vi "dialog_box for calibration.vi"(8 "error in (no error)":errorcluster caption="错误输入（无错误）") -> (0 "error out":errorcluster caption="错误输出", 2 "parameter for calibration out":T1, 3 "Cancelled?":bool caption="取消？")   [LabVIEW 2017]
doc: "该模板用于创建能够进行事件处理的对话框。"
uses:
  parameter set for calibration.ctl
panel:
  in  "磁铁位置":dbl=3.5
  in  "磁球大小（直径）":dbl=1.0
  in  "parameter for calibration":T1
  in  "校准步数":i32=20
  in  "首尾等待时间(s)":u32=1 caption="首尾I{卂时间(s)"
  in  "每步采样（frame）":u32=200
  in  "校准步长":dbl=0.1
  in  "分子长度（um）":dbl=1.0
  in  "Cancel":bool caption="取消"
  in  "OK":bool caption="确定"
  # "校准参数设置"
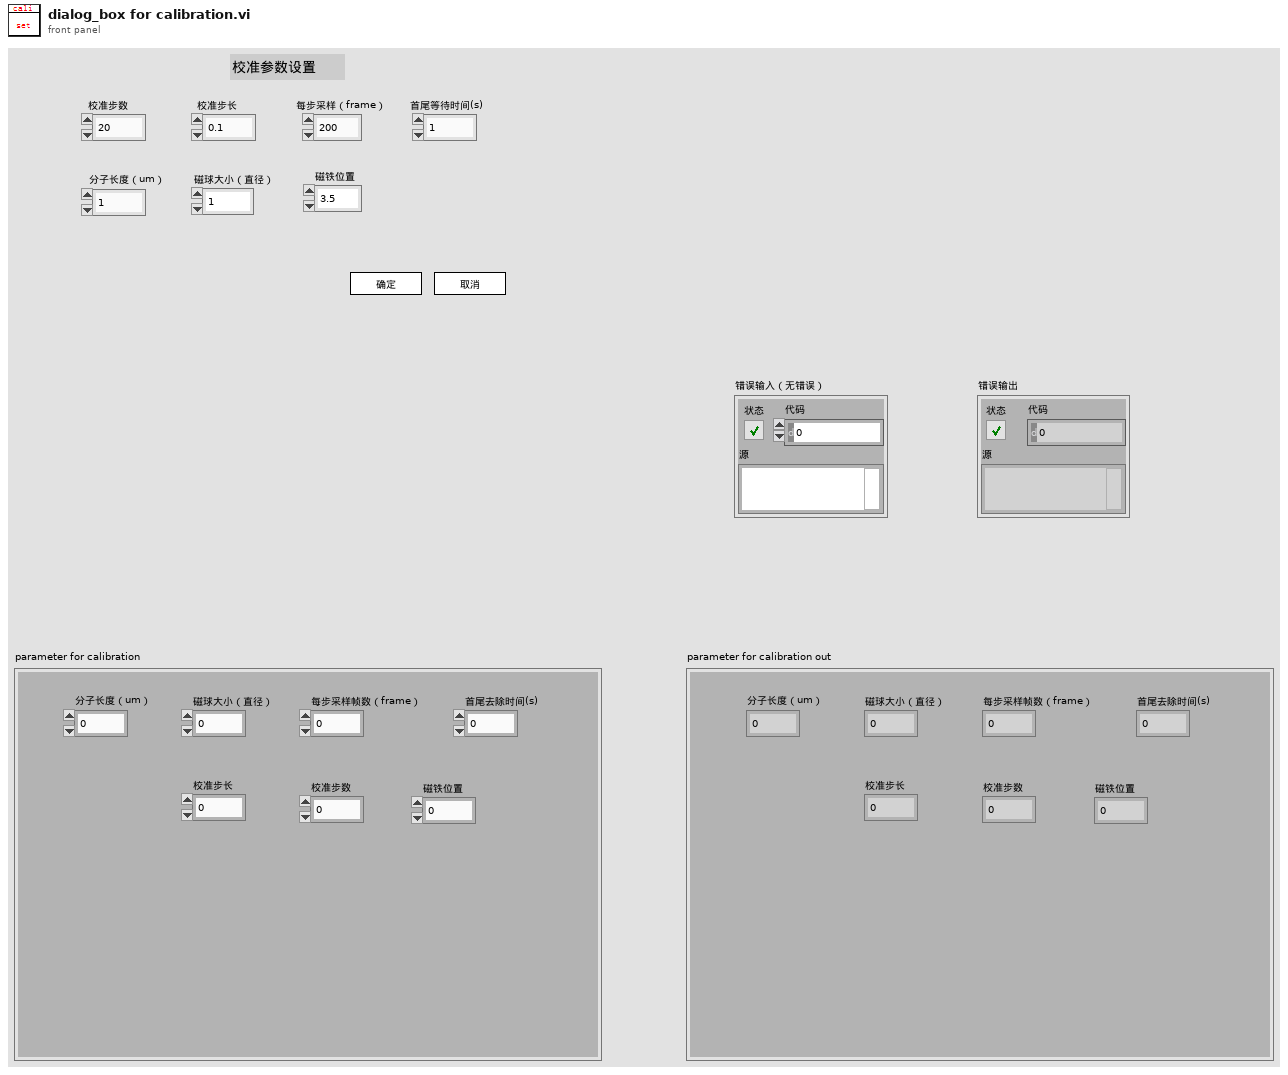
[diagram p1: front panel]
types:
  T1 = typedef "parameter set for calibration.ctl" = cluster{"分子长度（um）":dbl, "磁球大小（直径）":dbl, "校准步长":dbl, "每步采样帧数（frame）":u32, "首尾去除时间(s)":u32, "校准步数":i32, "磁铁位置":dbl}
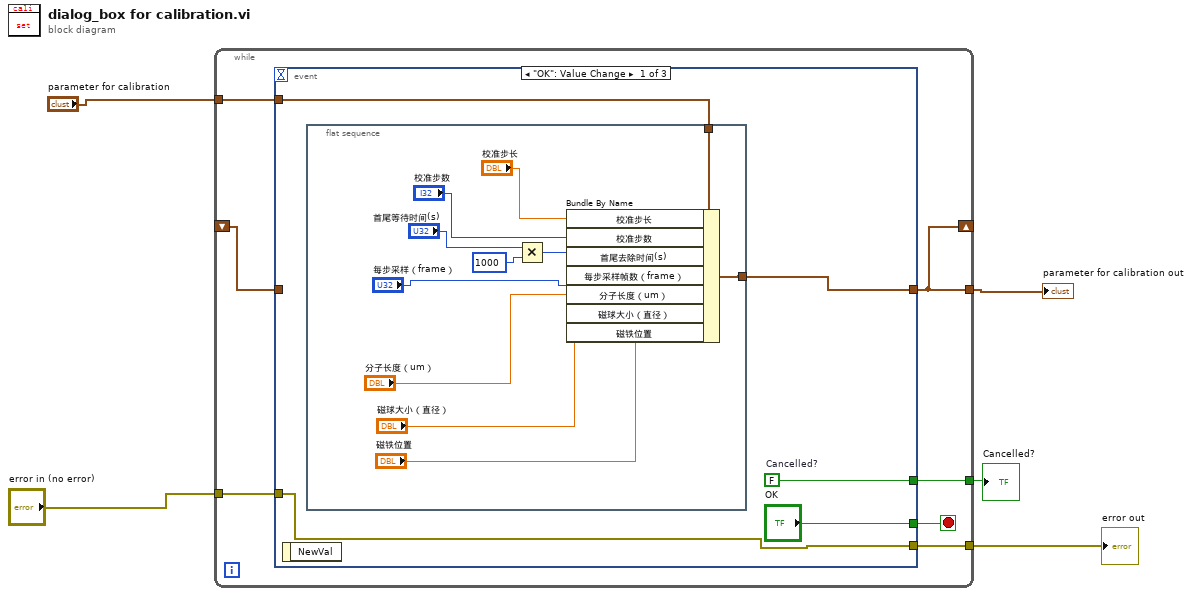
[diagram p0: block diagram]
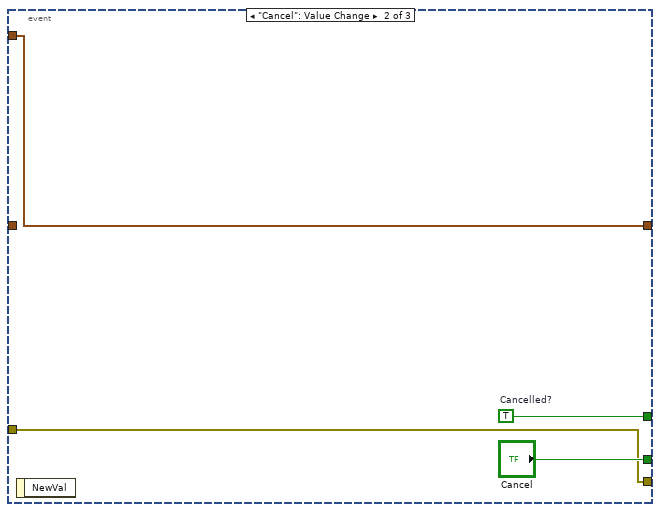
[diagram p2: hidden frame]
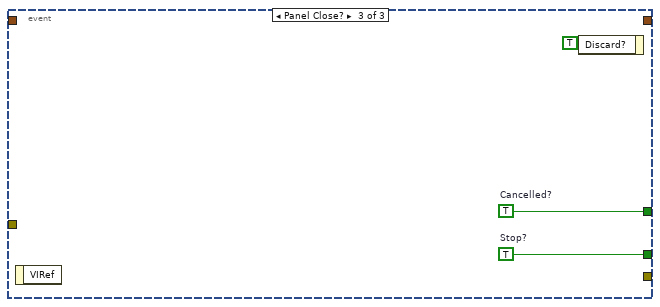
[diagram p3: hidden frame]
diagram:
  n1 = while {
    tunnel: [w11] -> w5
    tunnel: [w7] -> w4
    tunnel: "parameter for calibration" -> [w10]
    tunnel: "error in (no error)" -> [w9]
    tunnel: [w8] -> w2
    shift-right: [w7] -> _
    shift-left: _ -> [w6]
    stop <- w12 stop-if-true
    n2 = event shown="[0] \"OK\": Value Change" {
      selector: _ -> [_ _ _]
      dyn-events: _ -> [_ _ _]
      timeout: _ -> [_ _ _]
      tunnel: ["OK" "Cancel" w34] -> w12
      tunnel: [w17 w32 w33] -> w11
      tunnel: [w13 w29 _] -> w7
      tunnel: w10 -> [w14 w29 _]
      tunnel: [w15 w30 _] -> w8
      tunnel: w9 -> [w15 w30 _]
      tunnel: w6 -> [_ _ _]
      event "OK": Value Change {
        w17 = FALSE  # Cancelled?
        n3 = event-data() -> ()  [unwired: 1 in, 1 out]
        n4 = flat-sequence {
          tunnel: [w18] -> _
          tunnel: w14 -> [w19]
          tunnel: [w18] -> w13
          frame #0 {
            n5 = Multiply(x="首尾等待时间(s)", y=u32 1000) -> (x*y=w22:u32)
            n6 = Bundle By Name(cluster=w19, "校准步长"="校准步长", "校准步数"="校准步数", "首尾去除时间(s)"=w22, "每步采样帧数（frame）"="每步采样（frame）", "分子长度（um）"="分子长度（um）", "磁球大小（直径）"="磁球大小（直径）", "磁铁位置"="磁铁位置") -> (w18:T1)
          }
        }
      }
      event "Cancel": Value Change {
        w32 = TRUE  # Cancelled?
        n7 = event-data() -> ()  [unwired: 1 in, 1 out]
      }
      event Panel Close? {
        w33 = TRUE  # Cancelled?
        w34 = TRUE  # Stop?
        n8 = event-data() -> ()  [unwired: 1 in, 1 out]
        n9 = event-data("Discard?"=TRUE) -> ()  [unwired: 1 in, 1 out]
      }
    }
  }
  "Cancelled?" <- w5
  "parameter for calibration out" <- w4
  "error out" <- w2
